vi "RTM - Add Channels Updated.vi"(8 "error in (no error)":errorcluster, 11 "Node Ptr":u64 format="%.0x") -> (0 "error out":errorcluster)   [LabVIEW 2019, in "UDP-Custom-Device System Explorer.lvlib"]
uses:
  UDP-Custom-Device System Explorer.lvlib
  <vilib>/NI VeriStand/Custom Device API/Custom Device Item Ref.ctl
  <vilib>/NI VeriStand/Custom Device API/Custom Device Channel Type.ctl
  <vilib>/NI VeriStand/Custom Device API/Custom Device API.lvlib
  <vilib>/NI VeriStand/Custom Device Tools/Custom Device Utility Library/Custom Device Utility Library.lvlib
  Property Accessors/Shared Packet Accessors.lvlib
panel:
  in  "Remove":bool
  in  "Selected Channels":i32[](listbox)
  in  "Add":bool
  in  "Available Channels":string[](tree)
  in  "OK":bool
  in  "Cancel":bool
  in  "Initial Selection":T1[](array[typedef]) format="%.0x"
  in  "Tag":string
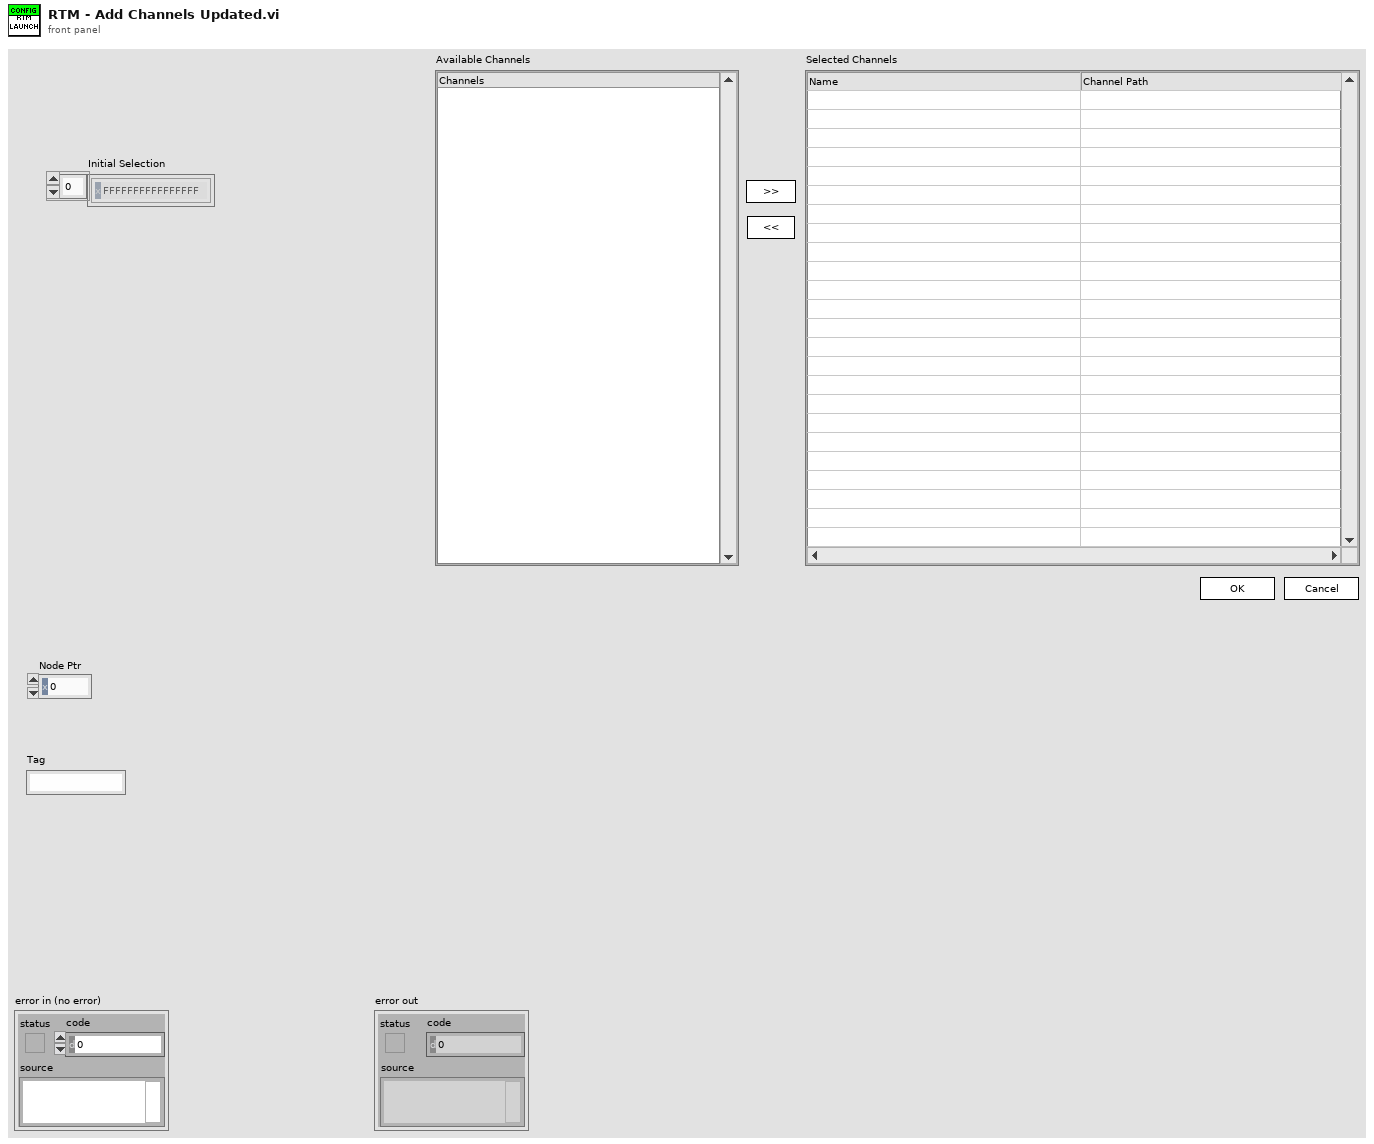
[diagram p1: front panel]
types:
  T1 = typedef "Custom Device API.lvlib/Custom Device Item Ref.ctl" = u64
  T2 = cluster{"Allow Section Selection (F)":bool, "Allow Multiple Selection (F)":bool}
  T3 = cluster{"Available Channels Label":string, "Selected Channels Label":string, "Mode":enum16{"Tx", "Rx"}}
  T4 = enum8{"Enabled", "Disabled", "Disabled and Grayed Out"}
  T5 = typedef "Custom Device API.lvlib/Custom Device Channel Type.ctl" = enum16{"Input", "Output"}
  T6 = typedef "LVRowAndColumnUnsignedTypeDef.ctl" = cluster{"Row":u32, "Column":u32}
  T7 = typedef "Custom Device API.lvlib/Custom Device Item Info.ctl" = cluster{"Name":string, "Is Channel":bool, "GUID":string, "Is Waveform":bool}
  T8 = typedef "Custom Device API.lvlib/Custom Device Channel.ctl" = cluster{"Type":T5, "Units":string, "Default Value":dbl, "Faultable":bool, "Scalable":bool}
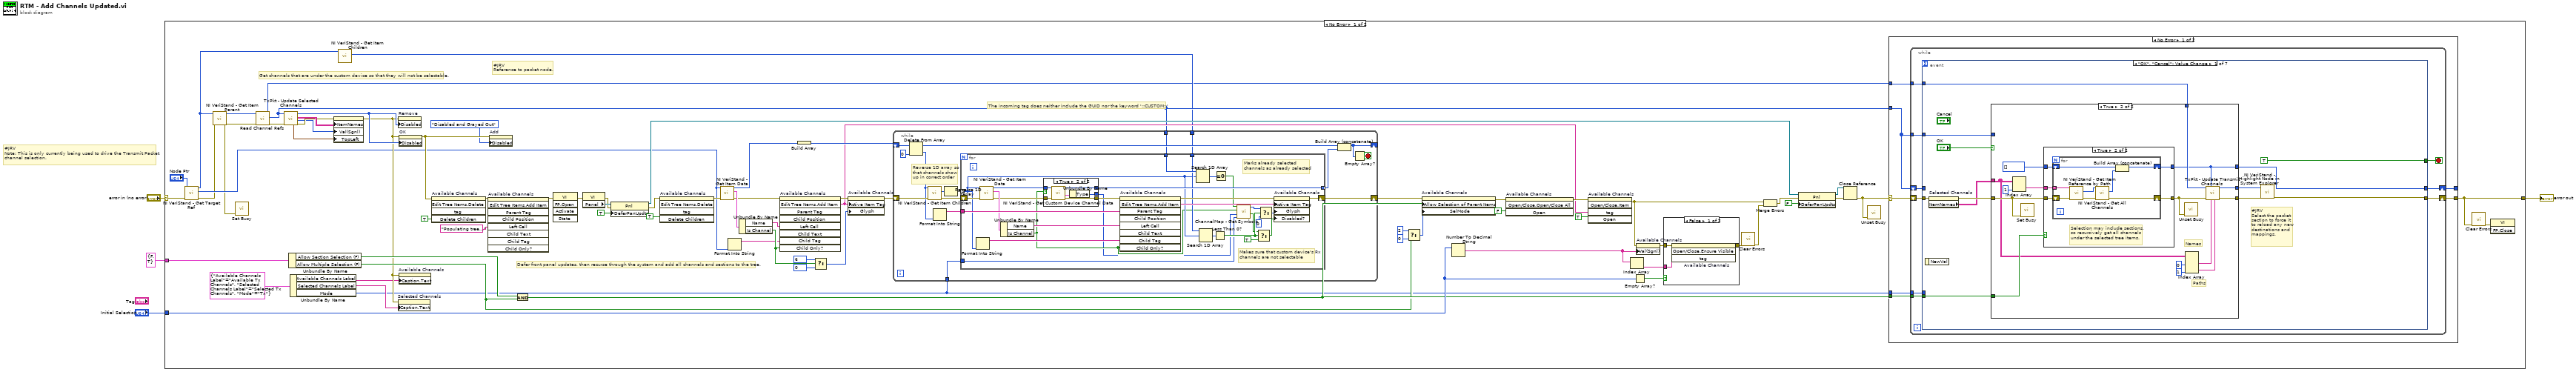
[diagram p0: block diagram]
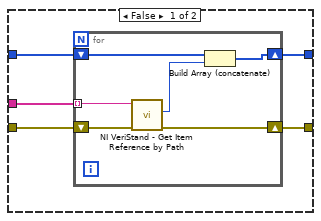
[diagram p4: hidden frame]
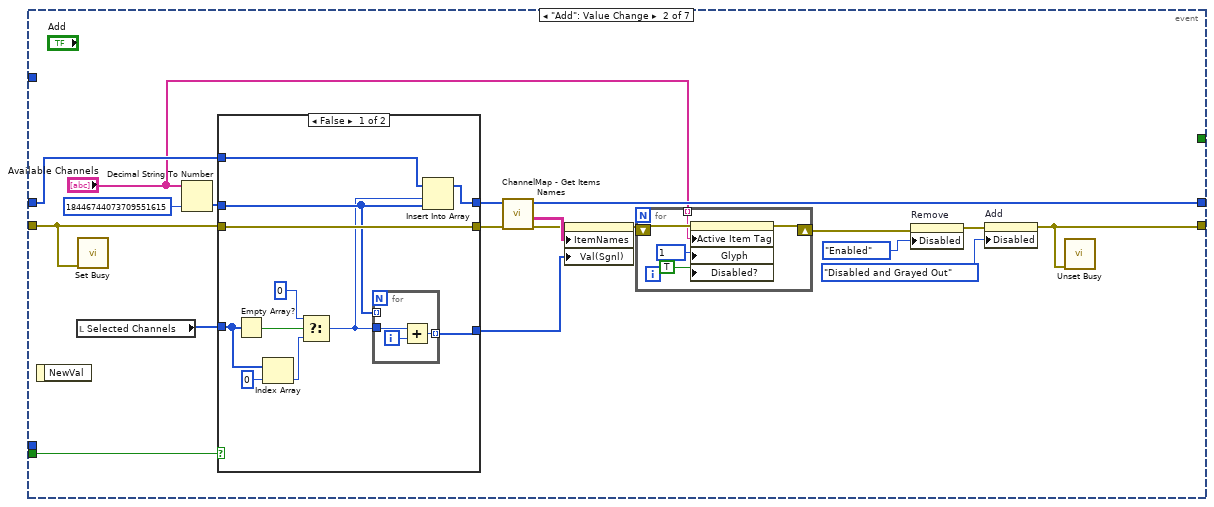
[diagram p5: hidden frame]
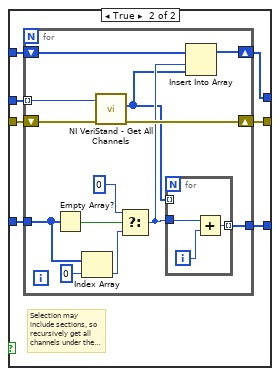
[diagram p6: hidden frame]
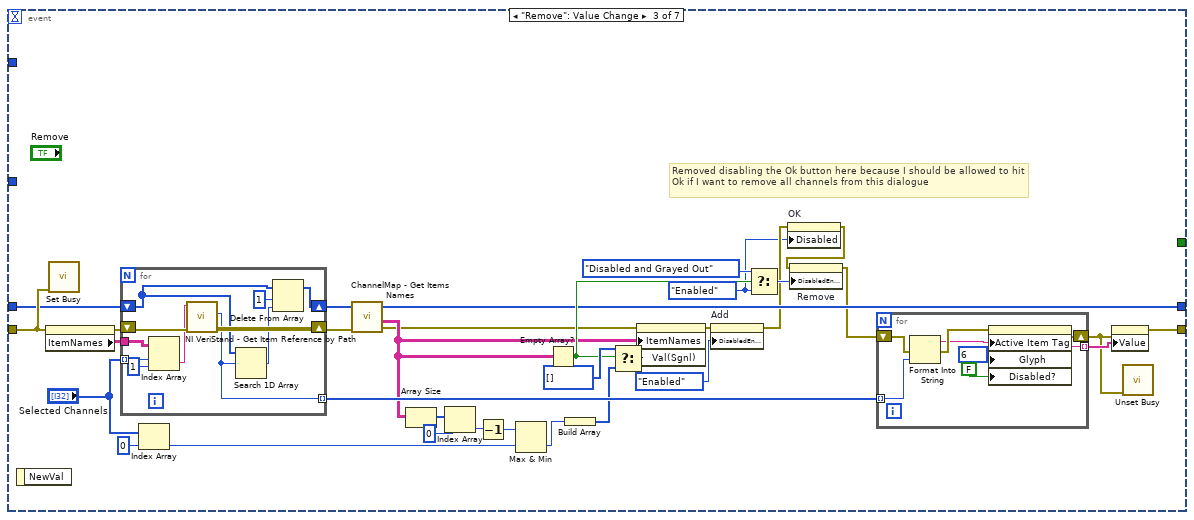
[diagram p7: hidden frame]
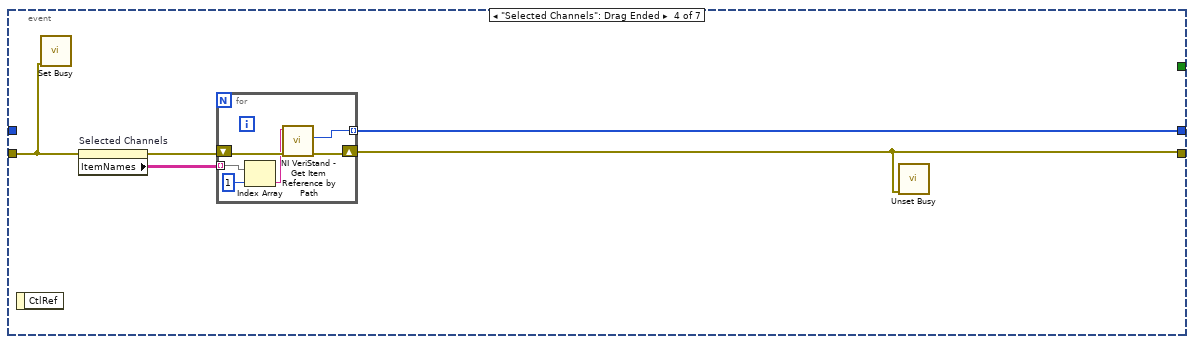
[diagram p8: hidden frame]
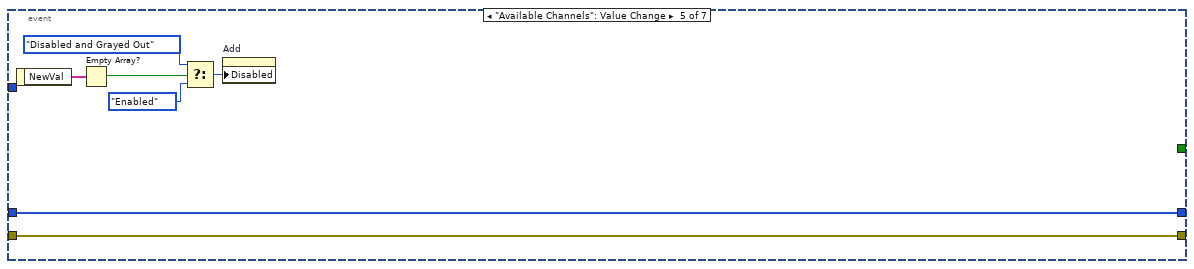
[diagram p9: hidden frame]
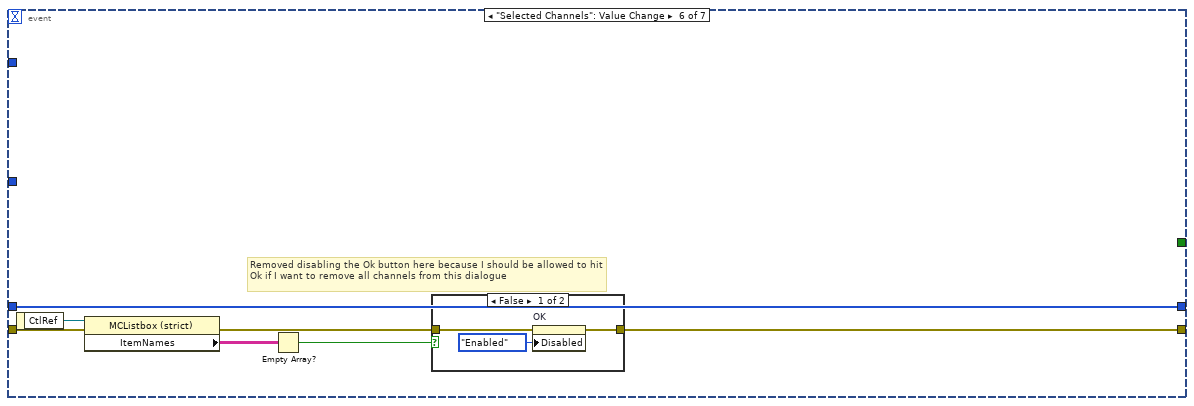
[diagram p10: hidden frame]
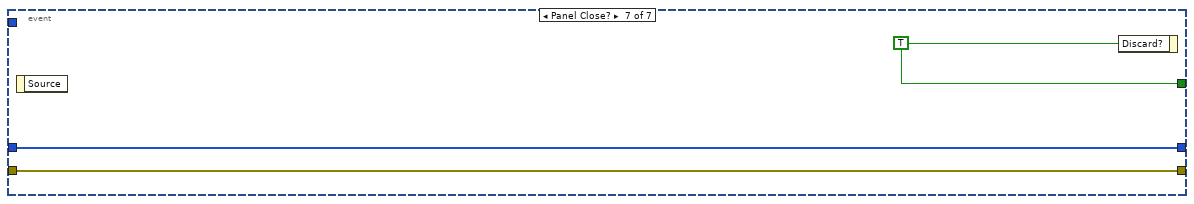
[diagram p12: hidden frame]
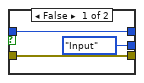
[diagram p14: hidden frame]
diagram:
  # "#JRV\nNote: This is only currently being used to drive the Transmit Packet\nchannel selection."
  # "The incoming tag does neither include the GUID nor the keyword '::CUSTOM::'"
  n1 = case shown="No Error" "error in (no error)" {
    selector: "error in (no error)" -> [w15 w352]
    tunnel: "Initial Selection" -> [w45 _]
    tunnel: [w63 w352] -> w1
    tunnel: T2 {"Allow Section Selection (F)"=FALSE, "Allow Multiple Selection (F)"=TRUE} ("Cluster") -> [w30 _]
    frame No Error {
      # "#JRV\nReference to packet node."
      # "Get channels that are under the custom device so that they will not be selectable."
      # "Defer front panel updates, then recurse through the system and add all channels and sections to the tree."
      n2 = call <vilib>:"NI VeriStand - Get Target Ref.vi"("error in"=w15, "Item Ref in"="Node Ptr") -> ("error out"=w12:errorcluster, "Target Ref"=w13:T1, "Item Ref out"=w9:T1)  [unwired: 6 in, 1 out]
      n3 = call <vilib>:"NI VeriStand - Get Item Parent.vi"("error in (no error)"=w12, "Item Ref in"=w9) -> ("error out"=w6:errorcluster, "Item Ref out"=w8:T1)  [unwired: 6 in, 2 out]
      n4 = call <vilib>:"Set Busy.vi"("error in (no error)"=w6) -> ()  [unwired: 3 in, 8 out]
      n5 = call "Read Channel Refs.vi"("error in (no error)"=w6, "Node Ptr"=w8) -> ("error out"=w16:errorcluster, "Dependent Node Refs"=w17:T1[], "Node Ptr out"=w7:T1)  [unwired: 7 in]
      n6 = call "TxPkt - Update Selected Channels.vi"("error in (no error)"=w16, "Dependent Node Refs"=w17) -> ("error out"=w26:errorcluster, "Val(Sgnl)"=w22:i32[], "Selected Channels"=w27:string[][], "Disabled Behavior"=w23:u8, "Top Left Visible Cell"=w11:T6)  [unwired: 5 in]
      n7 = Unbundle By Name(w30) -> ("Allow Section Selection (F)"=w29:bool, "Allow Multiple Selection (F)"=w28:bool)
      n8 = Unbundle By Name(T3 {"Available Channels Label"="Available Tx Channels", "Selected Channels Label"="Selected Tx Channels", "Mode"=enum."Tx"} ("Parameter")) -> ("Available Channels Label"=w20:string, "Selected Channels Label"=w19:string, "Mode"=w18:enum16{"Tx", "Rx"})
      n9 = property on="Selected Channels" class="MCListbox (strict)"(error in=w26, "ItemNames"=w27, "Val(Sgnl)"=w22, "TopLeft"=w11) -> (error out=w21:errorcluster)  [unwired: 1 in, 1 out]
      n10 = call <vilib>:"NI VeriStand - Get Item Children.vi"("Item Ref in"=w9) -> ("Child Refs"=w10:T1[])  [unwired: 7 in, 3 out]
      n11 = property on="Selected Channels" class="MCListbox (strict)"(error in=w21, "Caption.Text"=w19) -> ()  [unwired: 1 in, 2 out]
      n12 = property on="Remove" class="Bool"(error in=w21, "Disabled"=w23) -> ()  [unwired: 1 in, 2 out]
      n13 = property on="Available Channels" class="Tree (strict)"(error in=w21, "Caption.Text"=w20) -> ()  [unwired: 1 in, 2 out]
      n14 = property on="OK" class="Bool"(error in=w21, "Disabled"=w23) -> (error out=w25:errorcluster)  [unwired: 1 in, 1 out]
      n15 = invoke on="Available Channels" class="Tree (strict)" method="Edit Tree Items.Delete"(error in=w25, "Delete Children"=TRUE ("Delete Children?")) -> (error out=w79:errorcluster)  [unwired: 3 in, 4 out]
      n16 = invoke on="Available Channels" class="Tree (strict)" method="Edit Tree Items.Add Item"(error in=w79, "Left Cell"="Populating tree..." ("Tag")) -> (error out=w76:errorcluster)  [unwired: 7 in, 8 out]
      n17 = property on="Add" class="Bool"(error in=w25, "Disabled"=T4."Disabled and Grayed Out") -> ()  [unwired: 1 in, 2 out]
      n18 = Compound Arithmetic op=AND(w29, w28) -> (w32:bool)
      n19 = invoke class="VI" method="FP.Open"(error in=w76) -> (error out=w74:errorcluster)  [unwired: 4 in, 4 out]
      n20 = property class="VI"(error in=w74) -> (error out=w72:errorcluster, "Panel"=w73:refnum<vi>)  [unwired: 1 in, 1 out]
      n21 = property class="Pnl"(reference=w73, error in=w72, "DeferPanUpdts"=TRUE ("Defer Panel Updates")) -> (reference out=w66:refnum<vi>, error out=w70:errorcluster)
      n22 = invoke on="Available Channels" class="Tree (strict)" method="Edit Tree Items.Delete"(error in=w70, "Delete Children"=TRUE ("Delete Children?")) -> (error out=w50:errorcluster)  [unwired: 3 in, 4 out]
      n23 = call <vilib>:"NI VeriStand - Get Item Data.vi"("error in (no error)"=w50, "Item Ref in"=w13) -> ("error out"=w53:errorcluster, "Item Info"=w55:T7, "Item Ref out"=w51:T1)  [unwired: 7 out]
      n24 = Format Into String(w13) -> (resulting string=w54:string)  [unwired: 3 in, 1 out]
      n25 = Unbundle By Name(w55) -> ("Name"=w56:string, "Is Channel"=w60:bool)
      n26 = invoke on="Available Channels" class="Tree (strict)" method="Edit Tree Items.Add Item"(error in=w53, "Left Cell"=w56, "Child Tag"=w54, "Child Only?"=w60) -> (error out=w57:errorcluster, "Edit Tree Items:Add Item"=w36:string)  [unwired: 5 in, 7 out]
      n27 = Build Array(w51) -> (w69:T1[])
      n28 = Select(t=6, s=w60, f=0) -> (s? t:f=w61:i32)
      n29 = property on="Available Channels" class="Tree (strict)"(error in=w57, "Active Item Tag"=w36, "Glyph"=w61) -> (error out=w52:errorcluster)  [unwired: 1 in, 1 out]
      n30 = while {
        shift-right: [w305] -> w68
        shift-left: w52 -> [w311]
        shift-right: [w310] -> _
        shift-left: w69 -> [w314]
        tunnel: w17 -> [w302]
        tunnel: w18 -> [w301]
        tunnel: w10 -> [w300]
        stop <- w309 stop-if-true
        # "Reverse 1D array so that channels show up in correct order"
        n31 = Delete From Array(array=w314, index=0) -> (deleted portion=w304:T1, array with subset deleted=w312:T1[])  [unwired: 1 in]
        n32 = call <vilib>:"NI VeriStand - Get Item Children.vi"("error in (no error)"=w311, "Item Ref in"=w304) -> ("error out"=w308:errorcluster, "Child Refs"=w307:T1[])  [unwired: 8 out]
        n33 = Format Into String(w304) -> (resulting string=w303:string)  [unwired: 3 in, 1 out]
        n34 = Reverse 1D Array(array=w307) -> (reversed array=w299:T1[])
        n35 = for {
          shift-right: [w336] -> w305
          shift-left: w308 -> [w341]
          tunnel: w299 -> [w328] mode=indexing
          tunnel: [w333] -> w306 mode=indexing
          tunnel: w303 -> [w342]
          tunnel: w302 -> [w335]
          tunnel: w301 -> [w317]
          tunnel: w300 -> [w329]
          # "Marks already selected channels as already selected"
          # "Makes sure that custom device's Rx channels are not selectable"
          n36 = Format Into String(w328) -> (resulting string=w340:string)  [unwired: 3 in, 1 out]
          n37 = call <vilib>:"NI VeriStand - Get Item Data.vi"("error in (no error)"=w341, "Item Ref in"=w328) -> ("error out"=w332:errorcluster, "Item Info"=w339:T7, "Item Ref out"=w334:T1)  [unwired: 7 out]
          n38 = Unbundle By Name(w339) -> ("Name"=w330:string, "Is Channel"=w319:bool)
          n39 = case shown="True" w319 {
            tunnel: w334 -> [w345 w351]
            tunnel: [w345 w350] -> w333
            tunnel: w332 -> [w344 w349]
            tunnel: [w344 w348] -> w331
            tunnel: [Custom_Device_Channel_Type."Input" ("Type") w346] -> w318
            frame False {
            }
            frame True {
              n40 = call <vilib>:"NI VeriStand - Get Custom Device Channel Data.vi"("error in (no error)"=w349, "Channel Ref in"=w351) -> ("error out"=w348:errorcluster, "Channel"=w347:T8, "Channel Ref out"=w350:T1)  [unwired: 4 in, 3 out]
              n41 = Unbundle By Name(w347) -> ("Type"=w346:T5)
            }
          }
          n42 = invoke on="Available Channels" class="Tree (strict)" method="Edit Tree Items.Add Item"(error in=w331, "Parent Tag"=w342, "Left Cell"=w330, "Child Tag"=w340, "Child Only?"=w319) -> (error out=w338:errorcluster, "Edit Tree Items:Add Item"=w337:string)  [unwired: 4 in, 7 out]
          n43 = Search 1D Array(1D array=w335, element=w328) -> (index of element=w321:i32)  [unwired: 1 in]
          n44 = Search 1D Array(1D array=w329, element=w328) -> (index of element=w327:i32)  [unwired: 1 in]
          n45 = Less Than 0?(x=w327) -> (x < 0?=w323:bool)
          n46 = Greater Or Equal To 0?(x=w321) -> (x >= 0?=w320:bool)
          n47 = call "ChannelMap - Get Symbols.vi"("Mode"=w317, "Channel Type"=w318, "Is Channel?"=w319, "Is Selected?"=w320) -> ("Disabled?"=w315:bool, "Symbole"=w316:i32)  [unwired: 6 in]
          n48 = Select(t=w315, s=w323, f=TRUE) -> (s? t:f=w326:bool)
          n49 = Select(t=w316, s=w323, f=0) -> (s? t:f=w324:i32)
          n50 = property on="Available Channels" class="Tree (strict)"(error in=w338, "Active Item Tag"=w337, "Glyph"=w324, "Disabled?"=w326) -> (error out=w336:errorcluster)  [unwired: 1 in, 1 out]
        }
        n51 = Build Array (concatenate)(w312, w306) -> (w310:T1[])
        n52 = Empty Array?(array=w310) -> (empty?=w309:bool)
      }
      n53 = Select(t=2 ("Selection Mode"), s=w28, f=0 ("Selection Mode")) -> (s? t:f=w33:i32)
      n54 = property on="Available Channels" class="Tree (strict)"(error in=w68, "Allow Selection of Parent Items"=w32, "SelMode"=w33) -> (error out=w41:errorcluster)  [unwired: 1 in, 1 out]
      n55 = Number To Decimal String(number=w45) -> (decimal integer string=w43:string[])  [unwired: 1 out]
      n56 = invoke on="Available Channels" class="Tree (strict)" method="Open/Close.Open/Close All"(error in=w41, "Open"=FALSE ("Open?")) -> (error out=w39:errorcluster)  [unwired: 2 in, 3 out]
      n57 = invoke on="Available Channels" class="Tree (strict)" method="Open/Close.Item"(error in=w39, "tag"=w36, "Open"=TRUE ("Open?")) -> (error out=w37:errorcluster)  [unwired: 2 in, 4 out]
      n58 = Index Array(array=w43) -> (element=w42:string)  [unwired: 1 in]
      n59 = Empty Array?(array=w45) -> (empty?=w44:bool)
      n60 = property on="Available Channels" class="Tree (strict)"(error in=w37, "Val(Sgnl)"=w43) -> (error out=w47:errorcluster)  [unwired: 1 in, 1 out]
      n61 = case shown="False" w44 {
        tunnel: w47 -> [w82 w83]
        tunnel: [w81 w83] -> w46
        tunnel: w42 -> [w80 _]
        frame False {
          n62 = invoke on="Available Channels" class="Tree (strict)" method="Open/Close.Ensure Visible"(error in=w82, "tag"=w80) -> (error out=w81:errorcluster)  [unwired: 2 in, 3 out]
        }
        frame True {
        }
      }
      n63 = call <vilib>:"Clear Errors.vi"("error in (no error)"=w46) -> ("error out"=w49:errorcluster)  [unwired: 1 in, 5 out]
      n64 = Merge Errors(w37, w49) -> (w48:errorcluster)
      n65 = property class="Pnl"(reference=w66, error in=w48, "DeferPanUpdts"=FALSE ("Defer Panel Updates")) -> (reference out=w64:refnum<vi>, error out=w65:errorcluster)
      n66 = Close Reference(reference=w64, error in (no error)=w65) -> (error out=w31:errorcluster)
      n67 = call <vilib>:"Unset Busy.vi"("error in (no error)"=w31) -> ()  [unwired: 1 in, 10 out]
      n68 = case shown="No Error" w31 {
        selector: w31 -> [w90 w298]
        tunnel: [w89 w298] -> w63
        tunnel: [w88 w297] -> _
        tunnel: w32 -> [w87 _]
        tunnel: w17 -> [w86 w297]
        tunnel: w18 -> [w85 _]
        tunnel: w7 -> [w84 _]
        frame No Error {
          n69 = while {
            shift-right: [w98] -> w89
            shift-left: w90 -> [w99]
            tunnel: w87 -> [w96]
            shift-right: [w93] -> w88
            shift-left: w86 -> [w95]
            tunnel: w86 -> [w94]
            tunnel: w85 -> [w92]
            tunnel: w84 -> [w91]
            stop <- w97 stop-if-true
            n70 = event shown="[0] \"OK\", \"Cancel\": Value Change" {
              selector: _ -> [_ _ _ _ _ _ _]
              dyn-events: _ -> [_ _ _ _ _ _ _]
              timeout: _ -> [_ _ _ _ _ _ _]
              tunnel: w99 -> [w108 w170 w246 w269 w282 w287 w296]
              tunnel: [w104 w155 w219 w266 w282 w284 w296] -> w98
              tunnel: [TRUE ("Discard?") _ _ _ _ _ w295] -> w97
              tunnel: [w100 w166 w225 w265 w279 w289 w294] -> w93
              tunnel: w96 -> [w110 w169 _ _ _ _ _]
              tunnel: w95 -> [_ w168 w243 _ w279 w289 w294]
              tunnel: w94 -> [w106 _ _ _ _ _ _]
              tunnel: w92 -> [_ _ _ _ _ _ _]
              tunnel: w91 -> [w103 _ _ _ _ _ _]
              event "OK", "Cancel": Value Change {
                # "#JRV\nSelect the packet\nsection to force it\nto reload any new\ndestinations and\nmappings."
                n71 = event-data() -> ()  [unwired: 2 out]
                n72 = property on="Selected Channels" class="MCListbox (strict)"(error in=w108) -> (error out=w107:errorcluster, "ItemNames"=w105:string[][])  [unwired: 1 in, 1 out]
                n73 = case shown="True" "OK" {
                  tunnel: w105 -> [_ w122]
                  tunnel: w110 -> [_ w129]
                  tunnel: w107 -> [w114 w127]
                  tunnel: [w113 w120] -> w100
                  tunnel: [w114 w116] -> w101
                  tunnel: w106 -> [w113 _]
                  tunnel: w103 -> [w112 w121]
                  tunnel: [w112 w115] -> w102
                  frame False {
                  }
                  frame True {
                    # "Paths"
                    # "Names"
                    n74 = Index Array(array=w122, index (col)=1 ("disabled index (col)")) -> (element=w125:string[])  [unwired: 1 in]
                    n75 = call <vilib>:"Set Busy.vi"("error in (no error)"=w127) -> ()  [unwired: 3 in, 8 out]
                    n76 = case shown="True" w129 {
                      tunnel: w127 -> [w134 w145]
                      tunnel: [w130 w143] -> w120
                      tunnel: [w133 w142] -> w117
                      tunnel: T1[] [] ("Channel Refs") -> [w131 w144]
                      tunnel: w125 -> [w132 w141]
                      frame False {
                        n77 = for {
                          tunnel: w132 -> [w138] mode=indexing
                          shift-right: [w135] -> w130
                          shift-left: w131 -> [w136]
                          shift-right: [w139] -> w133
                          shift-left: w134 -> [w140]
                          n78 = call <vilib>:"NI VeriStand - Get Item Reference by Path.vi"("error in (no error)"=w140, "Item Path in"=w138) -> ("error out"=w139:errorcluster, "Item Ref"=w137:T1)  [unwired: 6 in, 2 out]
                          n79 = Build Array (concatenate)(w136, w137) -> (w135:T1[])
                        }
                      }
                      frame True {
                        # "Selection may include sections,\nso recursively get all channels\nunder the selected tree items."
                        n80 = for {
                          shift-right: [w151] -> w143
                          shift-left: w144 -> [w152]
                          shift-right: [w153] -> w142
                          shift-left: w145 -> [w148]
                          tunnel: w141 -> [w149] mode=indexing
                          n81 = call <vilib>:"NI VeriStand - Get Item Reference by Path.vi"("error in (no error)"=w148, "Item Path in"=w149) -> ("error out"=w147:errorcluster, "Item Ref"=w146:T1)  [unwired: 6 in, 2 out]
                          n82 = call <vilib>:"NI VeriStand - Get All Channels.vi"("error in"=w147, "Section Ref in"=w146) -> ("error out"=w153:errorcluster, "Channel Refs"=w150:T1[])  [unwired: 8 out]
                          n83 = Build Array (concatenate)(w152, w150) -> (w151:T1[])
                        }
                      }
                    }
                    n84 = call <vilib>:"Unset Busy.vi"("error in (no error)"=w117) -> ()  [unwired: 1 in, 10 out]
                    n85 = Index Array(array=w122, index (col) #1=0 ("disabled index (col)"), index (col) #2=1 ("index (col)")) -> (element #1=w119:string[], element #2=w118:string[])  [unwired: 2 in]
                    n86 = call "TxPkt - Update Transmit Channels.vi"("Channel Paths"=w118, "Channel Names"=w119, "Channle Node Refs"=w120, "error in (no error)"=w117, "Node Ptr"=w121) -> ("error out"=w116:errorcluster, "Node Ptr"=w115:T1)  [unwired: 5 in]
                  }
                }
                n87 = call <vilib>:"NI VeriStand - Highlight Node in System Explorer.vi"("error in (no error)"=w101, "Item Ref in"=w102) -> ("error out"=w104:errorcluster)  [unwired: 8 in, 1 out]
              }
              event "Add": Value Change {
                n88 = event-data() -> ()  [unwired: 2 out]
                n89 = local read "Selected Channels"() -> (w159:i32[])
                n90 = call <vilib>:"Set Busy.vi"("error in (no error)"=w170) -> ()  [unwired: 3 in, 8 out]
                n91 = Decimal String To Number(string="Available Channels", default (0L)=T1 18446744073709551615 ("Device Item Ref")) -> (number=w172:u64[])  [unwired: 2 out]
                n92 = case shown="False" w169 {
                  tunnel: w170 -> [w188 w198]
                  tunnel: [w185 w197] -> w167
                  tunnel: w172 -> [w180 w196]
                  tunnel: [w188 w195] -> w165
                  tunnel: w168 -> [w186 w194]
                  tunnel: w159 -> [w184 w193]
                  tunnel: [w178 w192] -> w158
                  frame False {
                    n93 = Empty Array?(array=w184) -> (empty?=w187:bool)
                    n94 = Index Array(array=w184, index=0) -> (element=w182:i32)
                    n95 = Select(t=0, s=w187, f=w182) -> (s? t:f=w179:i32)
                    n96 = for {
                      tunnel: w180 -> [_] mode=indexing
                      tunnel: w179 -> [w191]
                      tunnel: [w189] -> w178 mode=indexing
                      i -> [w190]
                      n97 = Add(x=w191, y=w190) -> (x+y=w189:i32)
                    }
                    n98 = Insert Into Array(array=w186, index=w179, new element=w180) -> (w185:T1[])
                  }
                  frame True {
                    # "Selection may include sections, so recursively get all channels under the selected tree items."
                    n99 = for {
                      shift-right: [w203] -> w197
                      shift-left: w194 -> [w202]
                      shift-right: [w210] -> w195
                      shift-left: w198 -> [w211]
                      tunnel: w196 -> [w209] mode=indexing
                      tunnel: w193 -> [w204]
                      tunnel: [w201] -> w192
                      n100 = Empty Array?(array=w204) -> (empty?=w205:bool)
                      n101 = Index Array(array=w204, index=0) -> (element=w207:i32)
                      n102 = call <vilib>:"NI VeriStand - Get All Channels.vi"("error in"=w211, "Section Ref in"=w209) -> ("error out"=w210:errorcluster, "Channel Refs"=w199:T1[])  [unwired: 8 out]
                      n103 = Select(t=0, s=w205, f=w207) -> (s? t:f=w200:i32)
                      n104 = for {
                        tunnel: w200 -> [w214]
                        tunnel: [w212] -> w201 mode=indexing
                        tunnel: w199 -> [_] mode=indexing
                        i -> [w213]
                        n105 = Add(x=w214, y=w213) -> (x+y=w212:i32)
                      }
                      n106 = Insert Into Array(array=w202, index=w200, new element=w199) -> (w203:T1[])
                    }
                  }
                }
                n107 = call "ChannelMap - Get Items Names.vi"("error IO 2"=w165, "TCP Channel Refs In"=w167) -> ("error IO"=w161:errorcluster, "Items Names"=w162:string[][], "TCP Channel Refs Out"=w166:T1[])  [unwired: 7 in]
                n108 = property on="Selected Channels" class="MCListbox (strict)"(error in=w161, "ItemNames"=w162, "Val(Sgnl)"=w158) -> (error out=w164:errorcluster)  [unwired: 1 in, 1 out]
                n109 = for {
                  shift-right: [w176] -> w157
                  shift-left: w164 -> [w177]
                  tunnel: "Available Channels" -> [w174] mode=indexing
                  n110 = property on="Available Channels" class="Tree (strict)"(error in=w177, "Active Item Tag"=w174, "Glyph"=1, "Disabled?"=TRUE ("Active Item:Disabled?")) -> (error out=w176:errorcluster)  [unwired: 1 in, 1 out]
                }
                n111 = property on="Remove" class="Bool"(error in=w157, "Disabled"=T4."Enabled") -> (error out=w156:errorcluster)  [unwired: 1 in, 1 out]
                n112 = property on="Add" class="Bool"(error in=w156, "Disabled"=T4."Disabled and Grayed Out") -> (error out=w155:errorcluster)  [unwired: 1 in, 1 out]
                n113 = call <vilib>:"Unset Busy.vi"("error in (no error)"=w155) -> ()  [unwired: 1 in, 10 out]
              }
              event "Remove": Value Change {
                w216 = T4."Enabled" ("Disabled")
                # "Removed disabling the Ok button here because I should be allowed to hit Ok if I want to remove all channels from this dialogue"
                n114 = event-data() -> ()  [unwired: 2 out]
                n115 = property on="Selected Channels" class="MCListbox (strict)"(error in=w246) -> (error out=w245:errorcluster, "ItemNames"=w244:string[][])  [unwired: 1 in, 1 out]
                n116 = call <vilib>:"Set Busy.vi"("error in (no error)"=w246) -> ()  [unwired: 3 in, 8 out]
                n117 = for {
                  tunnel: w244 -> [w255]
                  tunnel: "Selected Channels" -> [w256] mode=indexing
                  shift-right: [w254] -> w227
                  shift-left: w245 -> [w257]
                  shift-right: [w252] -> w224
                  shift-left: w243 -> [w253]
                  tunnel: [w249] -> w242 mode=indexing
                  n118 = Index Array(array=w255, index (row)=w256, index (col)=1 ("disabled index (col)")) -> (element=w247:string)
                  n119 = call <vilib>:"NI VeriStand - Get Item Reference by Path.vi"("error in (no error)"=w257, "Item Path in"=w247) -> ("error out"=w254:errorcluster, "Item Ref"=w249:T1)  [unwired: 6 in, 2 out]
                  n120 = Search 1D Array(1D array=w253, element=w249) -> (index of element=w250:i32)  [unwired: 1 in]
                  n121 = Delete From Array(array=w253, length=1, index=w250) -> (array with subset deleted=w252:T1[])  [unwired: 1 out]
                }
                n122 = Index Array(array="Selected Channels", index=0) -> (element=w230:i32)
                n123 = call "ChannelMap - Get Items Names.vi"("error IO 2"=w227, "TCP Channel Refs In"=w224) -> ("error IO"=w223:errorcluster, "Items Names"=w226:string[][], "TCP Channel Refs Out"=w225:T1[])  [unwired: 7 in]
                n124 = Array Size(array=w226) -> (size(s)=w234:i32[])
                n125 = Index Array(array=w234, index=0) -> (element=w232:i32)
                n126 = Decrement(x=w232) -> (x-1=w231:i32)
                n127 = Max & Min(x=w231, y=w230) -> (min(x,y)=w229:i32)  [unwired: 1 out]
                n128 = Empty Array?(array=w226) -> (empty?=w239:bool)
                n129 = Build Array(w229) -> (w236:i32[])
                n130 = Select(t=i32[] [] ("Selected TCP Channels"), s=w239, f=w236) -> (s? t:f=w240:i32[])
                n131 = property on="Selected Channels" class="MCListbox (strict)"(error in=w223, "ItemNames"=w226, "Val(Sgnl)"=w240) -> ()  [unwired: 1 in, 2 out]
                n132 = property on="Add" class="Bool"(error in=w223, "DisabledEnum"=T4."Enabled" ("Disabled")) -> (error out=w222:errorcluster)  [unwired: 1 in, 1 out]
                n133 = Select(t=T4."Disabled and Grayed Out" ("Disabled"), s=w239, f=w216) -> (s? t:f=w238:T4)
                n134 = property on="OK" class="Bool"(error in=w222, "Disabled"=w216) -> (error out=w221:errorcluster)  [unwired: 1 in, 1 out]
                n135 = property on="Remove" class="Bool"(error in=w221, "DisabledEnum"=w238) -> (error out=w220:errorcluster)  [unwired: 1 in, 1 out]
                n136 = for {
                  shift-right: [w262] -> w218
                  shift-left: w220 -> [w260]
                  tunnel: w242 -> [w261] mode=indexing
                  tunnel: [w258] -> w228 mode=indexing
                  n137 = Format Into String(error in=w260, w261) -> (resulting string=w258:string, error out=w259:errorcluster)  [unwired: 2 in]
                  n138 = property on="Available Channels" class="Tree (strict)"(error in=w259, "Active Item Tag"=w258, "Glyph"=6, "Disabled?"=FALSE ("Active Item:Disabled?")) -> (error out=w262:errorcluster)  [unwired: 1 in, 1 out]
                }
                n139 = property on="Available Channels" class="Tree (strict)"(error in=w218, "Value"=w228) -> (error out=w219:errorcluster)  [unwired: 1 in, 1 out]
                n140 = call <vilib>:"Unset Busy.vi"("error in (no error)"=w218) -> ()  [unwired: 1 in, 10 out]
              }
              event "Selected Channels": Drag Ended {
                n141 = event-data() -> ()  [unwired: 2 out]
                n142 = call <vilib>:"Set Busy.vi"("error in (no error)"=w269) -> ()  [unwired: 3 in, 8 out]
                n143 = property on="Selected Channels" class="MCListbox (strict)"(error in=w269) -> (error out=w268:errorcluster, "ItemNames"=w267:string[][])  [unwired: 1 in, 1 out]
                n144 = for {
                  tunnel: w267 -> [w274] mode=indexing
                  shift-right: [w273] -> w266
                  shift-left: w268 -> [w275]
                  tunnel: [w272] -> w265 mode=indexing
                  n145 = Index Array(array=w274, index=1 ("disabled index (col)")) -> (element=w271:string)
                  n146 = call <vilib>:"NI VeriStand - Get Item Reference by Path.vi"("error in (no error)"=w275, "Item Path in"=w271) -> ("error out"=w273:errorcluster, "Item Ref"=w272:T1)  [unwired: 6 in, 2 out]
                }
                n147 = call <vilib>:"Unset Busy.vi"("error in (no error)"=w266) -> ()  [unwired: 1 in, 10 out]
              }
              event "Available Channels": Value Change {
                n148 = event-data() -> ("NewVal"=w281:string[])  [unwired: 1 out]
                n149 = Empty Array?(array=w281) -> (empty?=w278:bool)
                n150 = Select(t=T4."Disabled and Grayed Out" ("Disabled"), s=w278, f=T4."Enabled" ("Disabled")) -> (s? t:f=w280:T4)
                n151 = property on="Add" class="Bool"("Disabled"=w280) -> ()  [unwired: 2 in, 2 out]
              }
              event "Selected Channels": Value Change {
                # "Removed disabling the Ok button here because I should be allowed to hit Ok if I want to remove all channels from this dialogue"
                n152 = event-data() -> ("CtlRef"=w288:refnum<vi>)  [unwired: 1 out]
                n153 = property class="MCListbox (strict)"(reference=w288, error in=w287) -> (error out=w285:errorcluster, "ItemNames"=w286:string[][])  [unwired: 1 out]
                n154 = Empty Array?(array=w286) -> (empty?=w283:bool)
                n155 = case shown="False" w283 {
                  tunnel: w285 -> [w292 w293]
                  tunnel: [w291 w293] -> w284
                  frame False {
                    n156 = property on="OK" class="Bool"(error in=w292, "Disabled"=T4."Enabled") -> (error out=w291:errorcluster)  [unwired: 1 in, 1 out]
                  }
                  frame True {
                  }
                }
              }
              event Panel Close? {
                w295 = TRUE ("Discard?")
                n157 = event-data() -> ()  [unwired: 2 out]
                n158 = event-data("Discard?"=w295) -> ()  [unwired: 1 in, 1 out]
              }
            }
          }
        }
        frame Error {
        }
      }
      n159 = call <vilib>:"Clear Errors.vi"("error in (no error)"=w63) -> ("error out"=w62:errorcluster)  [unwired: 1 in, 5 out]
      n160 = invoke class="VI" method="FP.Close"(error in=w62) -> ()  [unwired: 2 in, 3 out]
    }
    frame Error {
    }
  }
  "error out" <- w1
